vi "Auto Setup.vi"(8 "error in":errorcluster) -> ()   [LabVIEW 2019]
uses:
  <vilib>/Rock Robotics/WPI/DriverStation/WPI_DriverStationRobotMode2.ctl
  9a55a8d7-5b3f-4802-bfcc-96ea82079109.vi
  ed7fed8d-cbeb-403b-86f6-3c9ddeff16e0.vi
  <vilib>/Rock Robotics/Network Tables/NT Read String Array.vi
  Framework/Robot Global Data.vi
  <vilib>/Rock Robotics/Network Tables/NT Write Variant.vi
  <vilib>/Rock Robotics/Network Tables/NT Write String Array.vi
panel:
  out "error out":errorcluster
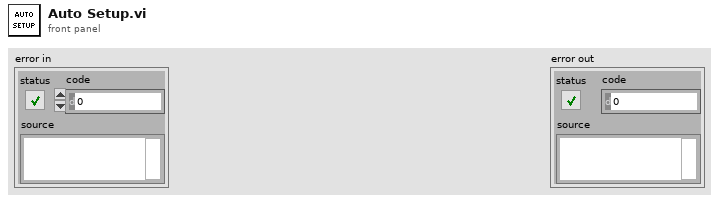
[diagram p1: front panel]
types:
  T1 = typedef "WPI_DriverStationRobotMode2.ctl" = enum16{"Autonomous Disabled", "Autonomous Enabled", "Teleop Disabled", "Teleop Enabled", "Disconnected", "Finish", "Test Disabled", "Test Enabled", "Emergency Stopped"}
  T2 = typedef "Single Cmd Info.ctl" = cluster{"Name":string, "CPTM.DataType":variant, "All Control Values Variant":cluster{"Name":string, "Variant Data":variant}[], "icon full":T3, "icon scaled":T3, "Path":path, "Subsystem Color":u32}
  T3 = typedef "imagedata.ctl" = cluster{"image type":i32, "image depth":i32, "image":u8[], "mask":u8[], "colors":u32[], "Rectangle":cluster{"left":i16, "top":i16, "right":i16, "bottom":i16}}
  T4 = typedef "Limits.ctl" = cluster{"Velocity (fps)":dbl, "Accel (fps^2)":dbl, "Jerk (fps^3)":dbl, "StoopidFast (fps)":dbl}
  T5 = cluster{"output cluster":cluster{"Reverse Path":bool, "Robot Backwards":bool}, "Trajectory Data":cluster{"Segment Name":string, "Type":enum16{"Accel Straight", "Const Straight", "Blend", "Circle"}, "Traj Pos Points":cluster{"x":dbl, "y":dbl, "th":dbl}[], "Traj Vel Points":cluster{"V":dbl, "th":dbl}[], "Accel Index":i32, "Decel Index":i32}[], cluster{"Time (s)":dbl, T2, bool}[], "output cluster":cluster{"Sample Period (s)":dbl, "Limits":T4, "Conditions":cluster{"vInitial (fps)":dbl, "vFinal (fps)":dbl}, cluster{dbl[], bool[]}}, "Updated Waypoints":cluster{"x":dbl, "y":dbl, "th":dbl}[], cluster{"Time (s)":dbl, "Distance (ft)":dbl}}
  T6 = cluster{"Segment Name":string, "Type":enum16{"Accel Straight", "Const Straight", "Blend", "Circle"}, "Traj Pos Points":cluster{"x":dbl, "y":dbl, "th":dbl}[], "Traj Vel Points":cluster{"V":dbl, "th":dbl}[], "Accel Index":i32, "Decel Index":i32}[]
  T7 = cluster{"Trajectory Data":cluster{"Segment Name":string, "Type":enum16{"Accel Straight", "Const Straight", "Blend", "Circle"}, "Traj Pos Points":cluster{"x":dbl, "y":dbl, "th":dbl}[], "Traj Vel Points":cluster{"V":dbl, "th":dbl}[], "Accel Index":i32, "Decel Index":i32}[], "Updated Waypoints":cluster{"x":dbl, "y":dbl, "th":dbl}[]}
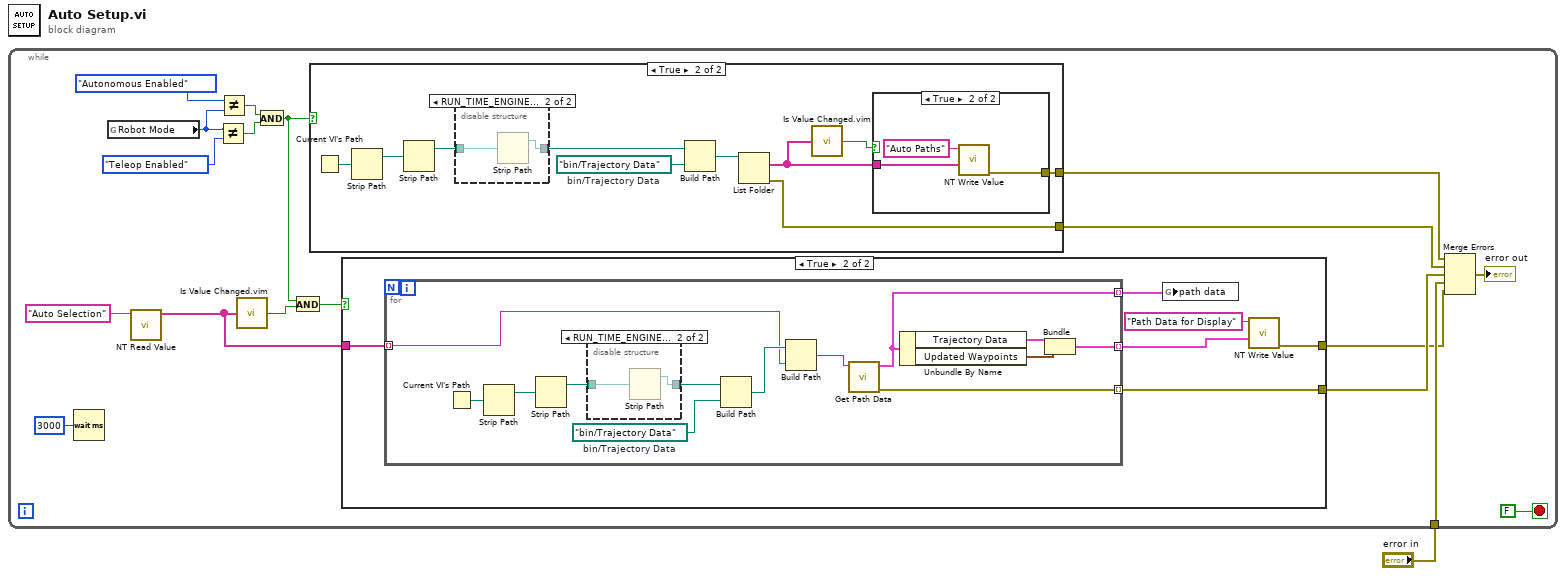
[diagram p0: block diagram]
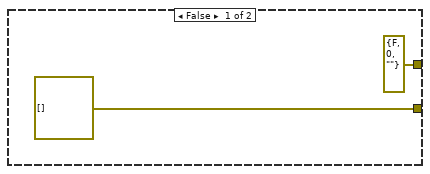
[diagram p2: hidden frame]
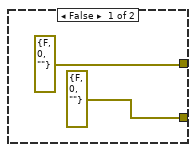
[diagram p4: hidden frame]
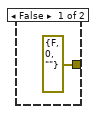
[diagram p5: hidden frame]
diagram:
  n1 = while {
    tunnel: "error in" -> [w6]
    stop <- FALSE stop-if-true
    n2 = Wait (ms)(milliseconds to wait=u32 3000) -> ()  [unwired: 1 out]
    n3 = global read "Robot Global Data.vi" "Robot Mode"() -> (w17:T1)
    n4 = call-poly <vilib>:"NT Read Value.vi"("Name"="Auto Selection") -> ("String Array"=w9:string[])  [unwired: 9 in, 1 out]
    n5 = Not Equal?(x=w17, y=WPI_DriverStationRobotMode2."Teleop Enabled") -> (x != y?=w14:bool)
    n6 = Not Equal?(x=WPI_DriverStationRobotMode2."Autonomous Enabled", y=w17) -> (x != y?=w15:bool)
    n7 = call "Is Value Changed.vim"("value"=w9) -> ("changed or first call?"=w10:bool)
    n8 = And(x=w15, y=w14) -> (x .and. y?=w13:bool)
    n9 = And(x=w13, y=w10) -> (x .and. y?=w12:bool)
    n10 = case shown="True" w13 {
      tunnel: [errorcluster {"status"=FALSE, "code"=0, "source"=""} ("error out") w49] -> w7
      tunnel: [errorcluster {"status"=FALSE, "code"=0, "source"=""} ("error out") w48] -> w4
      frame False {
      }
      frame True {
        w50 = path "bin/Trajectory Data"  # bin/Trajectory Data
        n11 = Current VI's Path() -> (path=w51:path)
        n12 = Strip Path(path=w51) -> (stripped path=w52:path)  [unwired: 1 out]
        n13 = Strip Path(path=w52) -> (stripped path=w54:path)  [unwired: 1 out]
        n14 = disable-structure shown="RUN_TIME_ENGINE==True, Default" {
          disable-tunnel: [w60 w61] -> w53
          disable-tunnel: w54 -> [w60 w62]
          frame condition #0 (active) {
          }
          frame condition #1 {
            n15 = Strip Path(path=w62) -> (stripped path=w61:path)  [unwired: 1 out]
          }
        }
        n16 = Build Path(base path=w53, name or relative path=w50) -> (appended path=w55:path)
        n17 = List Folder(path=w55) -> (filenames=w47:string[], error out=w49:errorcluster)  [unwired: 3 in, 2 out]
        n18 = call "Is Value Changed.vim"("value"=w47) -> ("changed or first call?"=w46:bool)
        n19 = case shown="True" w46 {
          tunnel: w47 -> [_ w58]
          tunnel: [errorcluster {"status"=FALSE, "code"=0, "source"=""} ("error out") w57] -> w48
          frame False {
          }
          frame True {
            n20 = call-poly <vilib>:"NT Write Value.vi"("String Array"=w58, "Name"="Auto Paths") -> ("error out"=w57:errorcluster)  [unwired: 9 in]
          }
        }
      }
    }
    n21 = case shown="True" w12 {
      tunnel: w9 -> [_ w27]
      tunnel: [errorcluster[] [] w26] -> w8
      tunnel: [errorcluster {"status"=FALSE, "code"=0, "source"=""} ("error out") w23] -> w3
      frame False {
      }
      frame True {
        n22 = for {
          tunnel: w27 -> [w34] mode=indexing
          tunnel: [w32] -> w26 mode=indexing
          tunnel: [w29] -> w24 mode=indexing
          tunnel: [w28] -> w22 mode=indexing
          w36 = path "bin/Trajectory Data"  # bin/Trajectory Data
          n23 = Current VI's Path() -> (path=w40:path)
          n24 = Strip Path(path=w40) -> (stripped path=w39:path)  [unwired: 1 out]
          n25 = Strip Path(path=w39) -> (stripped path=w37:path)  [unwired: 1 out]
          n26 = disable-structure shown="RUN_TIME_ENGINE==True, Default" {
            disable-tunnel: [w41 w42] -> w38
            disable-tunnel: w37 -> [w41 w43]
            frame condition #0 (active) {
            }
            frame condition #1 {
              n27 = Strip Path(path=w43) -> (stripped path=w42:path)  [unwired: 1 out]
            }
          }
          n28 = Build Path(base path=w38, name or relative path=w36) -> (appended path=w35:path)
          n29 = Build Path(base path=w35, name or relative path=w34) -> (appended path=w33:path)
          n30 = call "Get Path Data.vi"("Path"=w33) -> ("error out"=w32:errorcluster, "Path stuff"=w28:T5)  [unwired: 9 in]
          n31 = Unbundle By Name(w28) -> ("Trajectory Data"=w31:T6, "Updated Waypoints"=w30:cluster{"x":dbl, "y":dbl, "th":dbl}[])
          n32 = Bundle("Trajectory Data"=w31, "Updated Waypoints"=w30) -> (w29:T7)  [unwired: 1 in]
        }
        n33 = global write "Robot Global Data.vi" "path data"(w22) -> ()
        n34 = call-poly <vilib>:"NT Write Value.vi"("Variant"=w24, "Name"="Path Data for Display") -> ("error out"=w23:errorcluster)  [unwired: 9 in]
      }
    }
    n35 = Merge Errors(w4, w7, w8, w6, w3) -> (→"error out":errorcluster)
  }
